vi "Serial init.vi"(6 "controller":string, 8 "error in (no error)":errorcluster, 9 "errorLimit":u32, 10 "errorCounterIn":u32, 11 "VISA resource name":refnum<visa-resource-name>) -> (0 "error out":errorcluster, 1 "init":bool, 2 "errorCounterOut":u32, 3 "VISA resource name out":refnum<visa-resource-name>, 4 "error":string)   [LabVIEW 2018]
uses:
  <vilib>/Instr/_visa.llb/VISA Configure Serial Port (Instr).vi
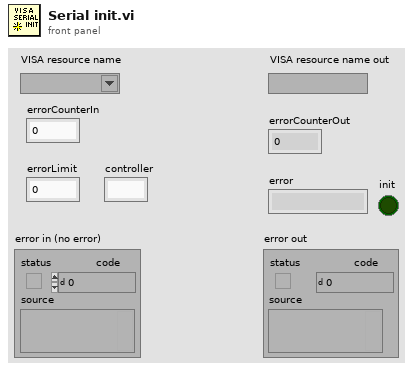
[diagram p1: front panel]
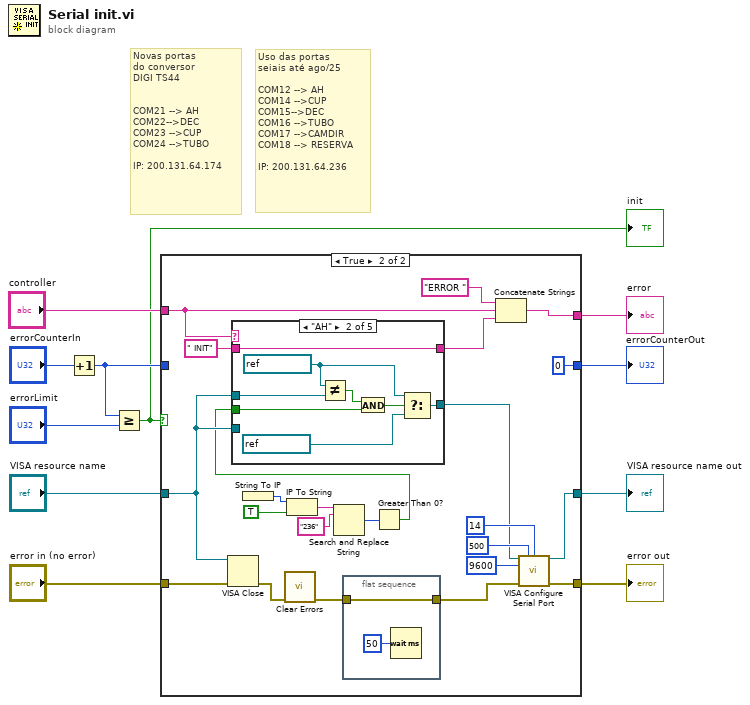
[diagram p0: block diagram]
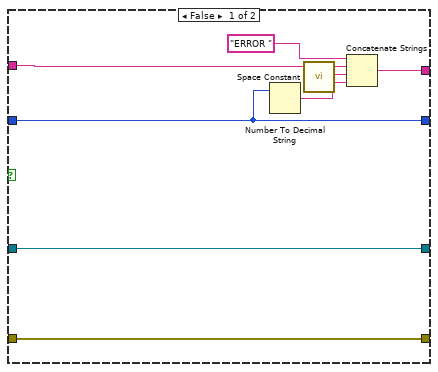
[diagram p2: hidden frame]
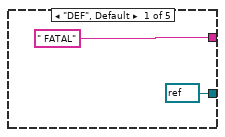
[diagram p3: hidden frame]
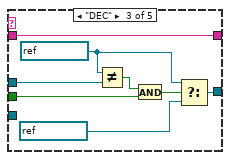
[diagram p4: hidden frame]
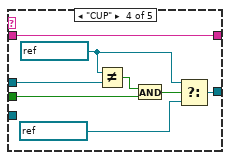
[diagram p5: hidden frame]
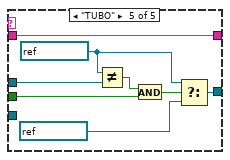
[diagram p6: hidden frame]
diagram:
  # "Uso das portas \nseiais até ago/25\n\nCOM12 --> AH\nCOM14 -->CUP\nCOM15-->DEC\nCOM16 -->TUBO\nCOM17 -->CAMDIR\nCOM18 --> RESERVA\n\nIP: 200.131.64.236"
  # "Novas portas\ndo conversor \nDIGI TS44\n\n\nCOM21 --> AH\nCOM22-->DEC\nCOM23 -->CUP\nCOM24 -->TUBO\n\nIP: 200.131.64.174"
  n1 = Increment(x="errorCounterIn") -> (x+1=w5:u32)
  n2 = Greater Or Equal?(x=w5, y="errorLimit") -> (x >= y?=w1:bool)
  "init" <- w1
  n3 = case shown="True" w1 {
    tunnel: [w19 w39] -> w11
    tunnel: "error in (no error)" -> [w19 w38]
    tunnel: [w17 w35] -> w9
    tunnel: "VISA resource name" -> [w17 w22]
    tunnel: w5 -> [w18 _]
    tunnel: [w18 u32 0] -> w4
    tunnel: [w16 w32] -> w3
    tunnel: "controller" -> [w14 w30]
    frame False {
      n4 = Number To Decimal String(number=w18) -> (decimal integer string=w13:string)  [unwired: 1 in]
      n5 = call <vilib>:"Space Constant.vi"() -> ("String"=w12:string)
      n6 = Concatenate Strings("ERROR ", w14, w12, w13) -> (w16:string)
    }
    frame True {
      n7 = VISA Close(VISA resource name=w22, error in (no error)=w38) -> (error out=w34:errorcluster)
      n8 = String To IP() -> (0:w25:u32)  [unwired: 1 in]
      n9 = call <vilib>:"Clear Errors.vi"("error in (no error)"=w34) -> ("error out"=w37:errorcluster)  [unwired: 5 in, 1 out]
      n10 = IP To String(1:TRUE ("dot notation? (F)"), 2:w25) -> (0:w26:string)
      n11 = Search and Replace String(input string=w26, search string="236") -> (number of replacements=w27:i32)  [unwired: 6 in, 3 out]
      n12 = flat-sequence {
        tunnel: w37 -> [w78]
        tunnel: [w78] -> w36
        frame #0 {
          n13 = Wait (ms)(milliseconds to wait=u32 50) -> ()  [unwired: 1 out]
        }
      }
      n14 = Greater Than 0?(x=w27) -> (x > 0?=w21:bool)
      n15 = case shown="\"AH\"" w30 {
        tunnel: " INIT" -> [_ w52 w60 w68 w76]
        tunnel: [" FATAL" w52 w60 w68 w76] -> w28
        tunnel: w22 -> [_ _ _ _ _]
        tunnel: w22 -> [_ w49 w57 w65 w73]
        tunnel: w21 -> [_ w48 w56 w64 w72]
        tunnel: [refnum<visa-resource-name> refnum ("VISA resource name") w45 w53 w61 w69] -> w20
        frame "DEF", Default {
        }
        frame "AH" {
          w50 = refnum<visa-resource-name> "COM12" ("VISA resource name")
          n16 = Not Equal?(x=w50, y=w49) -> (x != y?=w47:bool)
          n17 = And(x=w47, y=w48) -> (x .and. y?=w51:bool)
          n18 = Select(t=w50, s=w51, f=refnum<visa-resource-name> "COM21" ("VISA resource name")) -> (s? t:f=w45:refnum<visa-resource-name>)
        }
        frame "DEC" {
          w58 = refnum<visa-resource-name> "COM15" ("VISA resource name")
          n19 = Not Equal?(x=w58, y=w57) -> (x != y?=w55:bool)
          n20 = And(x=w55, y=w56) -> (x .and. y?=w59:bool)
          n21 = Select(t=w58, s=w59, f=refnum<visa-resource-name> "COM22" ("VISA resource name")) -> (s? t:f=w53:refnum<visa-resource-name>)
        }
        frame "CUP" {
          w66 = refnum<visa-resource-name> "COM14" ("VISA resource name")
          n22 = Not Equal?(x=w66, y=w65) -> (x != y?=w63:bool)
          n23 = And(x=w63, y=w64) -> (x .and. y?=w67:bool)
          n24 = Select(t=w66, s=w67, f=refnum<visa-resource-name> "COM23" ("VISA resource name")) -> (s? t:f=w61:refnum<visa-resource-name>)
        }
        frame "TUBO" {
          w74 = refnum<visa-resource-name> "COM16" ("VISA resource name")
          n25 = Not Equal?(x=w74, y=w73) -> (x != y?=w71:bool)
          n26 = And(x=w71, y=w72) -> (x .and. y?=w75:bool)
          n27 = Select(t=w74, s=w75, f=refnum<visa-resource-name> "COM24" ("VISA resource name")) -> (s? t:f=w69:refnum<visa-resource-name>)
        }
      }
      n28 = Concatenate Strings("ERROR ", w30, w28) -> (w32:string)
      n29 = call-poly "VISA Configure Serial Port"("VISA resource name"=w20, "timeout (10sec)"=u32 500 ("Tmo Value"), "termination char\n(0xA = '\\n' = LF)"=u8 14 ("termination char\n(0xA = '\\n' = LF)"), "baud rate (9600)"=u32 9600, "error in (no error)"=w36) -> ("VISA resource name out"=w35:refnum<visa-resource-name>, "error out"=w39:errorcluster)  [unwired: 9 in]
    }
  }
  "error out" <- w11
  "VISA resource name out" <- w9
  "errorCounterOut" <- w4
  "error" <- w3
